vi "Instantiate_llm_ollama.vi"(0 "model_name":string(combo)="tinyllama", 5 "Ollama URL":string="http://localhost:11434/", 7 "EnableStreaming":bool, 11 "error in (no error)":errorcluster) -> (4 "llm_ollama_chatmodels out":refnum<class "llm_ollama_chatmodels.lvclass">, 15 "error out":errorcluster)   [LabVIEW 2020, in "llm_ollama_chatmodels.lvclass"]
uses:
  llm_ollama_chatmodels.lvclass
  D:/Personal/LabVIEW LLMs/src/models/abstract_llm_base/abstract_llm_base.lvclass
  llm_ollama_chatmodels.lvclass/llm_ollama_chatmodels.ctl
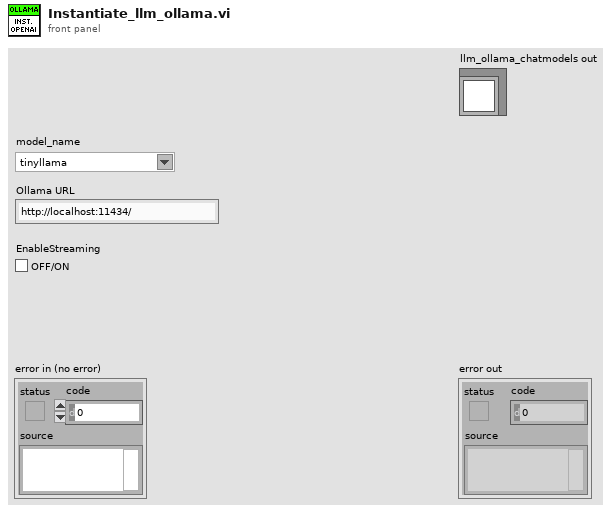
[diagram p1: front panel]
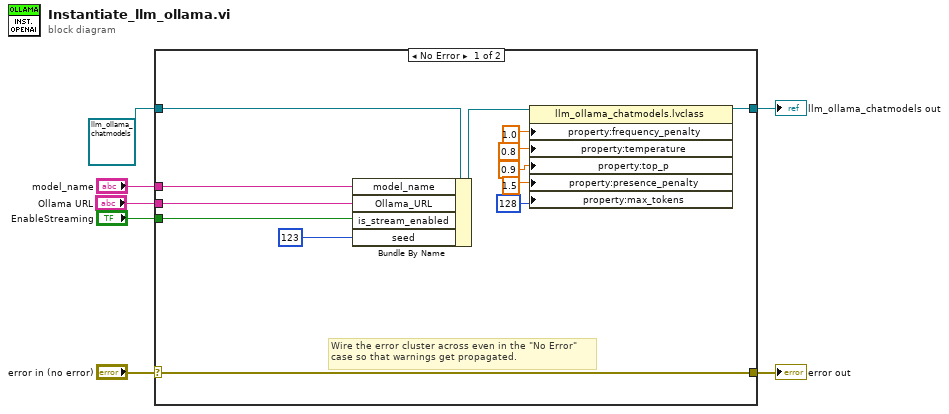
[diagram p0: block diagram]
diagram:
  n1 = case shown="No Error" "error in (no error)" {
    selector: "error in (no error)" -> [w20 w22]
    tunnel: [w20 w22] -> w6
    tunnel: [w14 w21] -> w4
    tunnel: refnum<class "llm_ollama_chatmodels.lvclass"> refnum ("llm_ollama_chatmodels in") -> [w19 w21]
    tunnel: "model_name" -> [w18 _]
    tunnel: "EnableStreaming" -> [w17 _]
    tunnel: "Ollama URL" -> [w16 _]
    frame No Error {
      # "Wire the error cluster across even in the \"No Error\"\ncase so that warnings get propagated."
      n2 = Bundle By Name(cluster=w19, "model_name"=w18, "Ollama_URL"=w16, "is_stream_enabled"=w17, "seed"=u32 123) -> (w15:refnum<class "llm_ollama_chatmodels.lvclass">)
      n3 = property class="llm_ollama_chatmodels.lvclass"(reference=w15, "property:frequency_penalty"=1.0 ("options.frequency_penalty"), "property:temperature"=0.8 ("options.temperature"), "property:top_p"=0.9 ("options.top_p"), "property:presence_penalty"=1.5 ("options.presence_penalty"), "property:max_tokens"=u32 128 ("max_tokens")) -> (reference out=w14:refnum<class "llm_ollama_chatmodels.lvclass">)  [unwired: 1 in, 1 out]
    }
    frame Error {
    }
  }
  "error out" <- w6
  "llm_ollama_chatmodels out" <- w4
